vi "Untitled 7 (SubVI) 1.vi"(0 "fraction core\nannihilations":dbl, 1 "Fermi angle\n   (mrad)":dbl, 5 "core width\n   (mrad)":dbl, 7 "sigma (mrad) in":dbl, 9 "1d - Acar":bool, 12 "collimator afstand\n       (mm)":dbl, 13 "spleetbreedte\n      (mm)":dbl) -> (2 "Array 5":dbl[](array[numeric]), 3 "Array 6":dbl[](array[numeric]), 4 "Array 4":i32[](array[numeric]), 6 "Numeric":i32, 8 "Array":dbl[](array[numeric]), 10 "Array 2":dbl[](array[numeric]), 14 "Array 3":dbl[](array[numeric]), 15 "Numeric 5":i32)   [LabVIEW 2013]
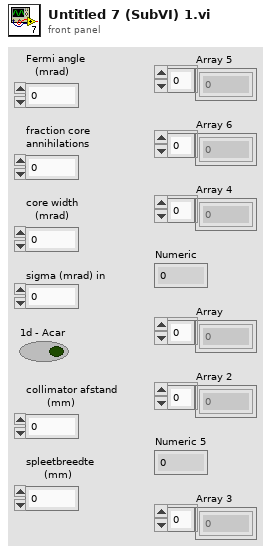
[diagram p1: front panel]
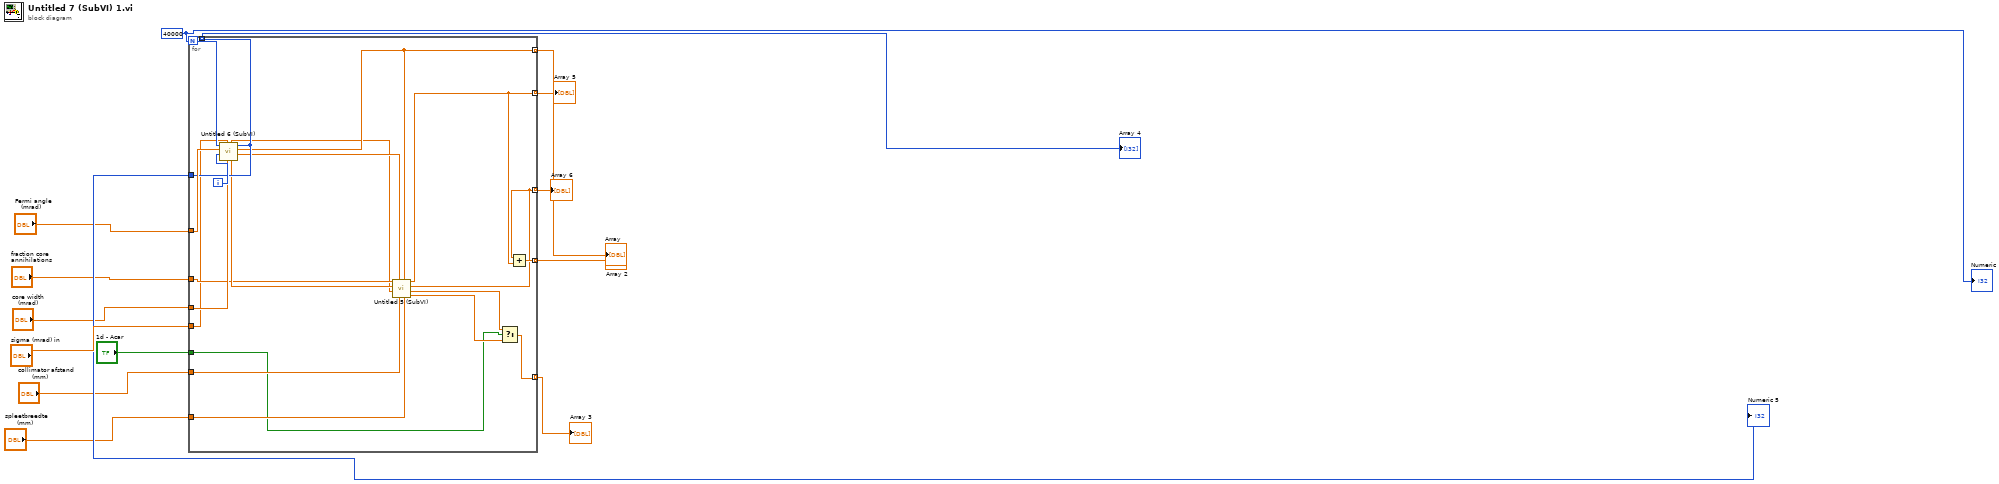
[diagram p0: block diagram]
diagram:
  w12 = 40000
  n1 = for {
    N: w12 -> [w34]
    tunnel: [w18] -> w14 mode=indexing
    tunnel: [w25] -> w1 mode=indexing
    tunnel: "Fermi angle\n   (mrad)" -> [w33]
    tunnel: [w29] -> w2 mode=indexing
    tunnel: "core width\n   (mrad)" -> [w32]
    tunnel: "fraction core\nannihilations" -> [w27]
    tunnel: [w31] -> w9 mode=indexing
    tunnel: "spleetbreedte\n      (mm)" -> [w23]
    tunnel: "collimator afstand\n       (mm)" -> [w24]
    tunnel: [w30] -> w7 mode=indexing
    tunnel: [w22] -> w8 mode=indexing
    tunnel: [w30] -> w11
    tunnel: "1d - Acar" -> [w19]
    tunnel: "sigma (mrad) in" -> [w17]
    i -> [w35]
    n2 = call "Untitled 6 (SubVI).vi"("core width\n   (mrad)"=w32, "sigma (mrad) in"=w17, "Numeric 7"=w35, "Fermi angle\n   (mrad)"=w33, "Numeric 6"=w34) -> ("Numeric 3"=w26:dbl, "Numeric 2"=w18:dbl, "Numeric 5"=w30:i32, "Numeric 4"=w28:dbl, "Numeric"=w16:dbl)  [unwired: 2 in]
    n3 = call "Untitled 5 (SubVI).vi"("spleetbreedte\n      (mm)"=w23, "Numeric 2"=w18, "collimator afstand\n       (mm)"=w24, "Numeric 6"=w26, "Numeric"=w16, "Numeric 7"=w28, "fraction core\nannihilations"=w27) -> ("Numeric 3"=w20:dbl, "Numeric 4"=w21:dbl, "Numeric 5"=w25:dbl, "Numeric 8"=w29:dbl)  [unwired: 1 in]
    n4 = Select(t=w21, s=w19, f=w20) -> (s? t:f=w22:dbl)
    n5 = Add(x=w25, y=w29) -> (x+y=w31:dbl)
  }
  "Array" <- w14
  "Numeric 5" <- w11
  "Array 2" <- w9
  "Array 3" <- w8
  "Array 4" <- w7
  "Array 5" <- w2
  "Array 6" <- w1
  "Numeric" <- w12
